vi "ReadCluster.vi"(1 "reference":refnum<vi>) -> (0 "Cluster":T6)   [LabVIEW 2013]
uses:
  <vilib>/Utility/miscctls.llb/LVBoundsTypeDef.ctl
  <vilib>/Utility/miscctls.llb/LVPositionTypeDef.ctl
  <vilib>/Utility/miscctls.llb/LVRectTypeDef.ctl
  <vilib>/Utility/miscctls.llb/LVDataSocketStatusTypeDef.ctl
  <vilib>/Utility/miscctls.llb/LVKeyNavTypeDef.ctl
panel:
  out "error out 72":errorcluster
  out "error out 71":errorcluster
  out "error out 70":errorcluster
  out "error out 69":errorcluster
  out "error out 68":errorcluster
  out "error out 67":errorcluster
  out "error out 66":errorcluster
  out "error out 65":errorcluster
  out "error out 64":errorcluster
  out "error out 63":errorcluster
  out "error out 62":errorcluster
  out "error out 61":errorcluster
  out "error out 60":errorcluster
  out "error out 59":errorcluster
  out "error out 58":errorcluster
  out "error out 57":errorcluster
  out "error out 56":errorcluster
  out "error out 55":errorcluster
  out "error out 54":errorcluster
  out "error out 53":errorcluster
  out "error out 52":errorcluster
  out "error out 51":errorcluster
  out "error out 50":errorcluster
  out "error out 49":errorcluster
  out "error out 48":errorcluster
  out "error out 47":errorcluster
  out "error out 46":errorcluster
  out "error out 45":errorcluster
  out "error out 44":errorcluster
  out "error out 43":errorcluster
  out "error out 42":errorcluster
  out "error out 41":errorcluster
  out "error out 40":errorcluster
  out "error out 39":errorcluster
  out "error out 38":errorcluster
  out "error out 37":errorcluster
  out "error out 36":errorcluster
  out "error out 35":errorcluster
  out "error out 34":errorcluster
  out "error out 33":errorcluster
  out "error out 32":errorcluster
  out "error out 31":errorcluster
  out "error out 30":errorcluster
  out "error out 29":errorcluster
  out "error out 28":errorcluster
  out "error out 27":errorcluster
  out "error out 26":errorcluster
  out "error out 25":errorcluster
  out "error out 24":errorcluster
  out "error out 23":errorcluster
  out "error out 22":errorcluster
  out "error out 21":errorcluster
  out "error out 20":errorcluster
  out "error out 19":errorcluster
  out "error out 18":errorcluster
  out "error out 17":errorcluster
  out "error out 16":errorcluster
  out "error out 15":errorcluster
  out "error out 14":errorcluster
  out "error out 13":errorcluster
  out "error out 12":errorcluster
  out "error out 11":errorcluster
  out "error out 10":errorcluster
  out "error out 9":errorcluster
  out "error out 8":errorcluster
  out "error out 7":errorcluster
  out "error out 6":errorcluster
  out "error out 5":errorcluster
  out "error out 4":errorcluster
  out "error out 3":errorcluster
  out "error out 2":errorcluster
  out "error out":errorcluster
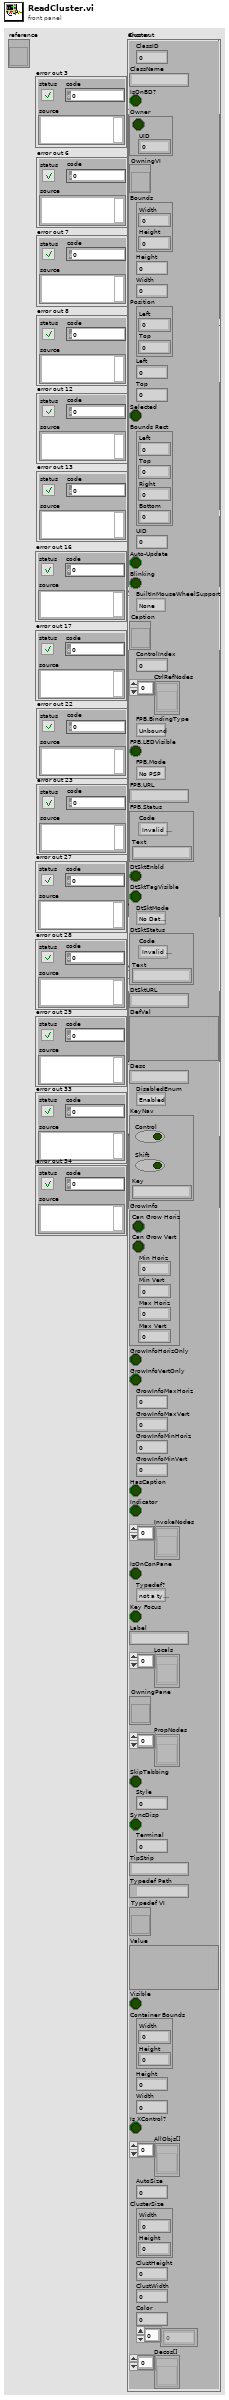
[diagram p1: front panel]
types:
  T1 = typedef "LVBoundsTypeDef.ctl" = cluster{"Width":u32, "Height":u32}
  T2 = typedef "LVPositionTypeDef.ctl" = cluster{"Left":i32, "Top":i32}
  T3 = typedef "LVRectTypeDef.ctl" = cluster{"Left":i16, "Top":i16, "Right":i16, "Bottom":i16}
  T4 = typedef "LVDataSocketStatusTypeDef.ctl" = cluster{"Code":enum32{"Invalid Status", "Unconnected", "Active", "Idle", "Error", "Connecting"}, "Text":string}
  T5 = typedef "LVKeyNavTypeDef.ctl" = cluster{"Control":bool, "Shift":bool, "Key":string}
  T6 = cluster{"ClassID":u32, "ClassName":string, "IsOnBD?":bool, "Owner":cluster{bool, "UID":i32}, "OwningVI":refnum<vi>, "Bounds":T1, "Height":u32, "Width":u32, "Position":T2, "Left":i32, "Top":i32, "Selected":bool, "Bounds Rect":T3, "UID":i32, "Auto-Update":bool, "Blinking":bool, "BuiltInMouseWheelSupport":enum16{"None", "On Hover", "On Key Focus", "On Hover or Key Focus"}, "Caption":refnum<vi>, "ControlIndex":i32, "CtrlRefNodes":refnum<vi>[], "FPB.BindingType":enum32{"Unbound", "Bound To PSP URL", "Bound To Variable Shortcut"}, "FPB.LEDVisible":bool, "FPB.Mode":enum32{"No PSP", "Read", "Write", "Write & Read"}, "FPB.URL":string, "FPB.Status":T4, "DtSktEnbld":bool, "DtSktTagVisible":bool, "DtSktMode":enum32{"No DataSocket", "Publish", "Subscribe", "Publish & Subscribe"}, "DtSktStatus":T4, "DtSktURL":string, "DefVal":variant, "Desc":string, "DisabledEnum":enum8{"Enabled", "Disabled", "Disabled and Grayed Out"}, "KeyNav":T5, "GrowInfo":cluster{"Can Grow Horiz":bool, "Can Grow Vert":bool, "Min Horiz":i16, "Min Vert":i16, "Max Horiz":i16, "Max Vert":i16}, "GrowInfoHorizOnly":bool, "GrowInfoVertOnly":bool, "GrowInfoMaxHoriz":i16, "GrowInfoMaxVert":i16, "GrowInfoMinHoriz":i16, "GrowInfoMinVert":i16, "HasCaption":bool, "Indicator":bool, "InvokeNodes":refnum<vi>[], "IsOnConPane":bool, "Typedef?":enum32{"not a typedef", "typedef", "strict typedef", "class private data"}, "Key Focus":bool, "Label":string, "Locals":refnum<vi>[], "OwningPane":refnum<vi>, "PropNodes":refnum<vi>[], "SkipTabbing":bool, "Style":u32, "SyncDisp":bool, "Terminal":i32, "TipStrip":string, "Typedef Path":path, "Typedef VI":refnum<vi>, "Value":variant, "Visible":bool, "Container Bounds":T1, "Height":u32, "Width":u32, "Is XControl?":bool, "AllObjs[]":refnum<vi>[], "AutoSize":u32, "ClusterSize":T1, "ClustHeight":u32, "ClustWidth":u32, "Color":u32, "Controls[]":i32[], "Decos[]":refnum<vi>[]}
  T7 = enum16{"None", "On Hover", "On Key Focus", "On Hover or Key Focus"}
  T8 = enum32{"No PSP", "Read", "Write", "Write & Read"}
  T9 = enum32{"Unbound", "Bound To PSP URL", "Bound To Variable Shortcut"}
  T10 = enum32{"No DataSocket", "Publish", "Subscribe", "Publish & Subscribe"}
  T11 = enum8{"Enabled", "Disabled", "Disabled and Grayed Out"}
  T12 = enum32{"not a typedef", "typedef", "strict typedef", "class private data"}
  T13 = cluster{"Can Grow Horiz":bool, "Can Grow Vert":bool, "Min Horiz":i16, "Min Vert":i16, "Max Horiz":i16, "Max Vert":i16}
  T14 = cluster{"ClassID":u32, "ClassName":string, "IsOnBD?":bool, "Cluster":cluster{bool, "UID":i32}, "OwningVI":refnum<vi>, "Bounds":T1, "Height":u32, "Width":u32, "Position":T2, "Left":i32, "Top":i32, "Selected":bool, "Bounds Rect":T3, "UID":i32, "Auto-Update":bool, "Blinking":bool, "BuiltInMouseWheelSupport":enum16{"None", "On Hover", "On Key Focus", "On Hover or Key Focus"}, "Caption":refnum<vi>, "ControlIndex":i32, "CtrlRefNodes":refnum<vi>[], "FPB.BindingType":enum32{"Unbound", "Bound To PSP URL", "Bound To Variable Shortcut"}, "FPB.LEDVisible":bool, "FPB.Mode":enum32{"No PSP", "Read", "Write", "Write & Read"}, "FPB.URL":string, "FPB.Status":T4, "DtSktEnbld":bool, "DtSktTagVisible":bool, "DtSktMode":enum32{"No DataSocket", "Publish", "Subscribe", "Publish & Subscribe"}, "DtSktStatus":T4, "DtSktURL":string, "DefVal":variant, "Desc":string, "DisabledEnum":enum8{"Enabled", "Disabled", "Disabled and Grayed Out"}, "KeyNav":T5, "GrowInfo":cluster{"Can Grow Horiz":bool, "Can Grow Vert":bool, "Min Horiz":i16, "Min Vert":i16, "Max Horiz":i16, "Max Vert":i16}, "GrowInfoHorizOnly":bool, "GrowInfoVertOnly":bool, "GrowInfoMaxHoriz":i16, "GrowInfoMaxVert":i16, "GrowInfoMinHoriz":i16, "GrowInfoMinVert":i16, "HasCaption":bool, "Indicator":bool, "InvokeNodes":refnum<vi>[], "IsOnConPane":bool, "Typedef?":enum32{"not a typedef", "typedef", "strict typedef", "class private data"}, "Key Focus":bool, "Text":string, "Locals":refnum<vi>[], "OwningPane":refnum<vi>, "PropNodes":refnum<vi>[], "SkipTabbing":bool, "Style":u32, "SyncDisp":bool, "UID":i32, "TipStrip":string, "Typedef Path":path, "Typedef VI":refnum<vi>, "Value":variant, "Visible":bool, "Container Bounds":T1, "Height":u32, "Width":u32, "Is XControl?":bool, "AllObjs[]":refnum<vi>[], "AutoSize":u32, "ClusterSize":T1, "ClustHeight":u32, "ClustWidth":u32, "Color":u32, i32[], "Decos[]":refnum<vi>[]}
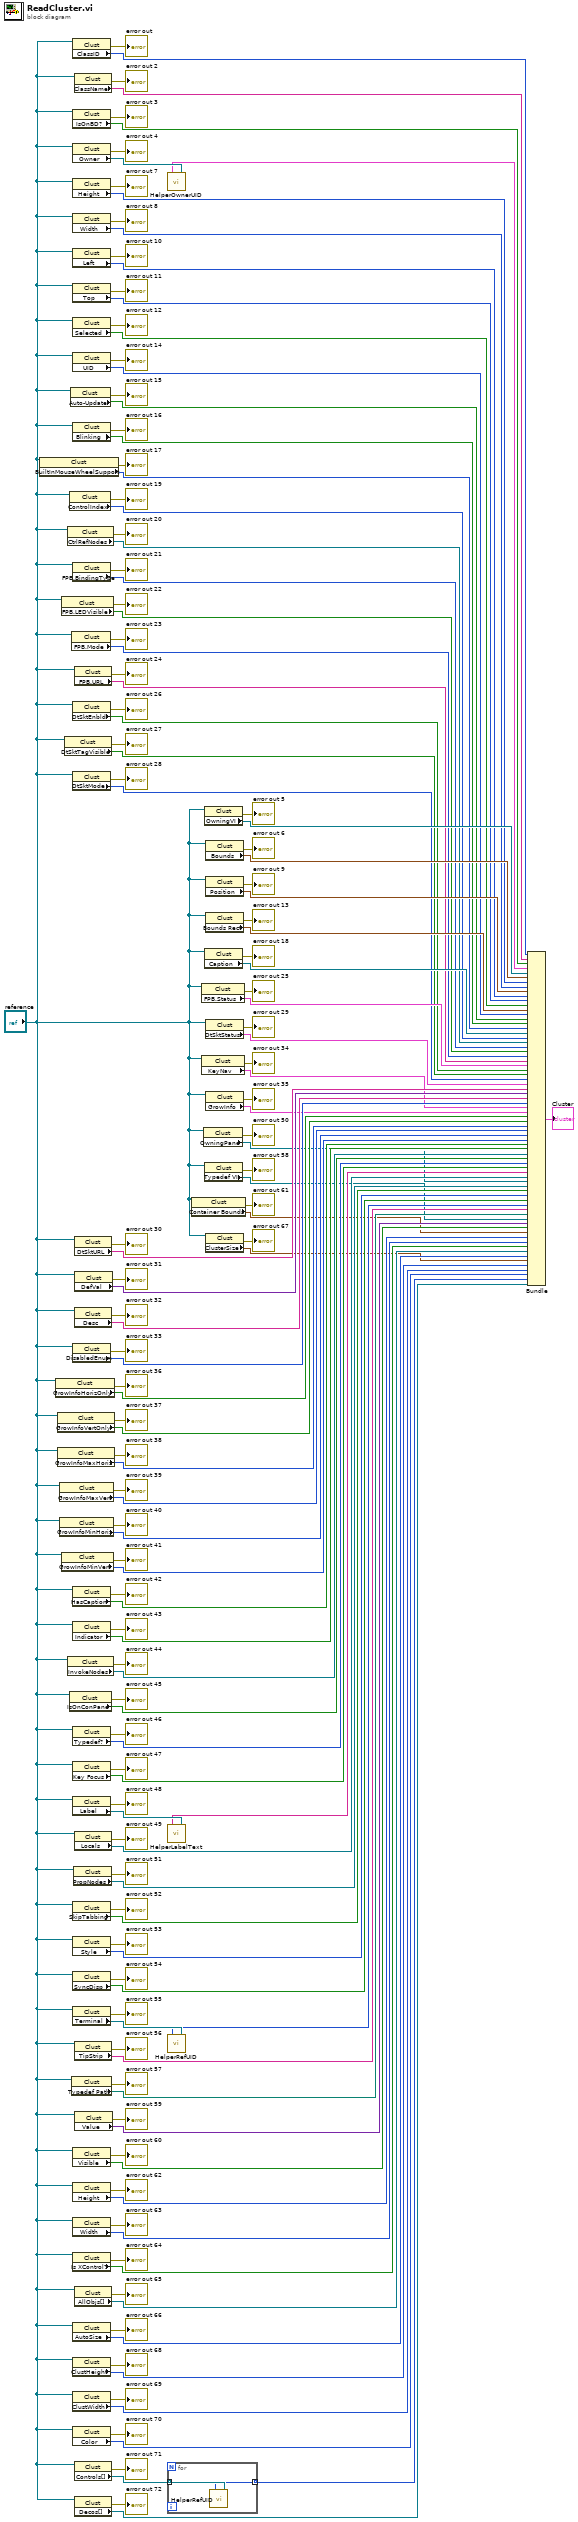
[diagram p0: block diagram]
diagram:
  n1 = property class="Clust"(reference="reference") -> (error out=→"error out 17":errorcluster, "BuiltInMouseWheelSupport"=w115:T7)  [unwired: 1 in, 1 out]
  n2 = property class="Clust"(reference="reference") -> (error out=→"error out 36":errorcluster, "GrowInfoHorizOnly"=w77:bool)  [unwired: 1 in, 1 out]
  n3 = property class="Clust"(reference="reference") -> (error out=→"error out 37":errorcluster, "GrowInfoVertOnly"=w75:bool)  [unwired: 1 in, 1 out]
  n4 = property class="Clust"(reference="reference") -> (error out=→"error out 38":errorcluster, "GrowInfoMaxHoriz"=w73:i16)  [unwired: 1 in, 1 out]
  n5 = property class="Clust"(reference="reference") -> (error out=→"error out 39":errorcluster, "GrowInfoMaxVert"=w71:i16)  [unwired: 1 in, 1 out]
  n6 = property class="Clust"(reference="reference") -> (error out=→"error out 40":errorcluster, "GrowInfoMinHoriz"=w69:i16)  [unwired: 1 in, 1 out]
  n7 = property class="Clust"(reference="reference") -> (error out=→"error out 22":errorcluster, "FPB.LEDVisible"=w105:bool)  [unwired: 1 in, 1 out]
  n8 = property class="Clust"(reference="reference") -> (error out=→"error out 41":errorcluster, "GrowInfoMinVert"=w67:i16)  [unwired: 1 in, 1 out]
  n9 = property class="Clust"(reference="reference") -> (error out=→"error out 27":errorcluster, "DtSktTagVisible"=w95:bool)  [unwired: 1 in, 1 out]
  n10 = property class="Clust"(reference="reference") -> (error out=→"error out 20":errorcluster, "CtrlRefNodes"=w109:refnum<vi>[])  [unwired: 1 in, 1 out]
  n11 = property class="Clust"(reference="reference") -> (error out=→"error out 44":errorcluster, "InvokeNodes"=w61:refnum<vi>[])  [unwired: 1 in, 1 out]
  n12 = property class="Clust"(reference="reference") -> (error out=→"error out 45":errorcluster, "IsOnConPane"=w59:bool)  [unwired: 1 in, 1 out]
  n13 = property class="Clust"(reference="reference") -> (error out=→"error out 19":errorcluster, "ControlIndex"=w111:i32)  [unwired: 1 in, 1 out]
  n14 = property class="Clust"(reference="reference") -> (error out=→"error out 15":errorcluster, "Auto-Update"=w119:bool)  [unwired: 1 in, 1 out]
  n15 = property class="Clust"(reference="reference") -> (error out=→"error out 23":errorcluster, "FPB.Mode"=w103:T8)  [unwired: 1 in, 1 out]
  n16 = property class="Clust"(reference="reference") -> (error out=→"error out 57":errorcluster, "Typedef Path"=w33:path)  [unwired: 1 in, 1 out]
  n17 = property class="Clust"(reference="reference") -> (error out=→"error out":errorcluster, "ClassID"=w148:u32)  [unwired: 1 in, 1 out]
  n18 = property class="Clust"(reference="reference") -> (error out=→"error out 3":errorcluster, "IsOnBD?"=w144:bool)  [unwired: 1 in, 1 out]
  n19 = property class="Clust"(reference="reference") -> (error out=→"error out 4":errorcluster, "Owner"=w142:refnum<vi>)  [unwired: 1 in, 1 out]
  n20 = property class="Clust"(reference="reference") -> (error out=→"error out 7":errorcluster, "Height"=w135:u32)  [unwired: 1 in, 1 out]
  n21 = property class="Clust"(reference="reference") -> (error out=→"error out 8":errorcluster, "Width"=w133:u32)  [unwired: 1 in, 1 out]
  n22 = property class="Clust"(reference="reference") -> (error out=→"error out 10":errorcluster, "Left"=w129:i32)  [unwired: 1 in, 1 out]
  n23 = property class="Clust"(reference="reference") -> (error out=→"error out 11":errorcluster, "Top"=w127:i32)  [unwired: 1 in, 1 out]
  n24 = property class="Clust"(reference="reference") -> (error out=→"error out 12":errorcluster, "Selected"=w125:bool)  [unwired: 1 in, 1 out]
  n25 = property class="Clust"(reference="reference") -> (error out=→"error out 14":errorcluster, "UID"=w121:i32)  [unwired: 1 in, 1 out]
  n26 = property class="Clust"(reference="reference") -> (error out=→"error out 16":errorcluster, "Blinking"=w117:bool)  [unwired: 1 in, 1 out]
  n27 = property class="Clust"(reference="reference") -> (error out=→"error out 21":errorcluster, "FPB.BindingType"=w107:T9)  [unwired: 1 in, 1 out]
  n28 = property class="Clust"(reference="reference") -> (error out=→"error out 26":errorcluster, "DtSktEnbld"=w97:bool)  [unwired: 1 in, 1 out]
  n29 = property class="Clust"(reference="reference") -> (error out=→"error out 28":errorcluster, "DtSktMode"=w93:T10)  [unwired: 1 in, 1 out]
  n30 = property class="Clust"(reference="reference") -> (error out=→"error out 33":errorcluster, "DisabledEnum"=w83:T11)  [unwired: 1 in, 1 out]
  n31 = property class="Clust"(reference="reference") -> (error out=→"error out 42":errorcluster, "HasCaption"=w65:bool)  [unwired: 1 in, 1 out]
  n32 = property class="Clust"(reference="reference") -> (error out=→"error out 43":errorcluster, "Indicator"=w63:bool)  [unwired: 1 in, 1 out]
  n33 = property class="Clust"(reference="reference") -> (error out=→"error out 46":errorcluster, "Typedef?"=w57:T12)  [unwired: 1 in, 1 out]
  n34 = property class="Clust"(reference="reference") -> (error out=→"error out 47":errorcluster, "Key Focus"=w55:bool)  [unwired: 1 in, 1 out]
  n35 = property class="Clust"(reference="reference") -> (error out=→"error out 48":errorcluster, "Label"=w53:refnum<vi>)  [unwired: 1 in, 1 out]
  n36 = property class="Clust"(reference="reference") -> (error out=→"error out 52":errorcluster, "SkipTabbing"=w44:bool)  [unwired: 1 in, 1 out]
  n37 = property class="Clust"(reference="reference") -> (error out=→"error out 53":errorcluster, "Style"=w42:u32)  [unwired: 1 in, 1 out]
  n38 = property class="Clust"(reference="reference") -> (error out=→"error out 54":errorcluster, "SyncDisp"=w40:bool)  [unwired: 1 in, 1 out]
  n39 = property class="Clust"(reference="reference") -> (error out=→"error out 55":errorcluster, "Terminal"=w38:refnum<vi>)  [unwired: 1 in, 1 out]
  n40 = property class="Clust"(reference="reference") -> (error out=→"error out 60":errorcluster, "Visible"=w27:bool)  [unwired: 1 in, 1 out]
  n41 = property class="Clust"(reference="reference") -> (error out=→"error out 62":errorcluster, "Height"=w23:u32)  [unwired: 1 in, 1 out]
  n42 = property class="Clust"(reference="reference") -> (error out=→"error out 63":errorcluster, "Width"=w21:u32)  [unwired: 1 in, 1 out]
  n43 = property class="Clust"(reference="reference") -> (error out=→"error out 64":errorcluster, "Is XControl?"=w19:bool)  [unwired: 1 in, 1 out]
  n44 = property class="Clust"(reference="reference") -> (error out=→"error out 66":errorcluster, "AutoSize"=w15:u32)  [unwired: 1 in, 1 out]
  n45 = property class="Clust"(reference="reference") -> (error out=→"error out 68":errorcluster, "ClustHeight"=w11:u32)  [unwired: 1 in, 1 out]
  n46 = property class="Clust"(reference="reference") -> (error out=→"error out 69":errorcluster, "ClustWidth"=w9:u32)  [unwired: 1 in, 1 out]
  n47 = property class="Clust"(reference="reference") -> (error out=→"error out 70":errorcluster, "Color"=w7:u32)  [unwired: 1 in, 1 out]
  n48 = property class="Clust"(reference="reference") -> (error out=→"error out 51":errorcluster, "PropNodes"=w46:refnum<vi>[])  [unwired: 1 in, 1 out]
  n49 = property class="Clust"(reference="reference") -> (error out=→"error out 2":errorcluster, "ClassName"=w146:string)  [unwired: 1 in, 1 out]
  n50 = property class="Clust"(reference="reference") -> (error out=→"error out 24":errorcluster, "FPB.URL"=w101:string)  [unwired: 1 in, 1 out]
  n51 = property class="Clust"(reference="reference") -> (error out=→"error out 30":errorcluster, "DtSktURL"=w89:string)  [unwired: 1 in, 1 out]
  n52 = property class="Clust"(reference="reference") -> (error out=→"error out 32":errorcluster, "Desc"=w85:string)  [unwired: 1 in, 1 out]
  n53 = property class="Clust"(reference="reference") -> (error out=→"error out 49":errorcluster, "Locals"=w50:refnum<vi>[])  [unwired: 1 in, 1 out]
  n54 = property class="Clust"(reference="reference") -> (error out=→"error out 56":errorcluster, "TipStrip"=w35:string)  [unwired: 1 in, 1 out]
  n55 = property class="Clust"(reference="reference") -> (error out=→"error out 65":errorcluster, "AllObjs[]"=w17:refnum<vi>[])  [unwired: 1 in, 1 out]
  n56 = property class="Clust"(reference="reference") -> (error out=→"error out 71":errorcluster, "Controls[]"=w5:refnum<vi>[])  [unwired: 1 in, 1 out]
  n57 = property class="Clust"(reference="reference") -> (error out=→"error out 72":errorcluster, "Decos[]"=w2:refnum<vi>[])  [unwired: 1 in, 1 out]
  n58 = property class="Clust"(reference="reference") -> (error out=→"error out 31":errorcluster, "DefVal"=w87:variant)  [unwired: 1 in, 1 out]
  n59 = property class="Clust"(reference="reference") -> (error out=→"error out 59":errorcluster, "Value"=w29:variant)  [unwired: 1 in, 1 out]
  n60 = call "HelperOwnerUID.vi"("Generic in"=w142) -> ("Cluster"=w141:cluster{bool, "UID":i32})
  n61 = call "HelperLabelText.vi"("Text in"=w53) -> ("Text"=w52:string)
  n62 = call "HelperRefUID.vi"("Text in"=w38) -> ("UID"=w37:i32)
  n63 = for {
    tunnel: w5 -> [w152] mode=indexing
    tunnel: [w151] -> w4 mode=indexing
    n64 = call "HelperRefUID.vi"("Text in"=w152) -> ("UID"=w151:i32)
  }
  n65 = property class="Clust"(reference="reference") -> (error out=→"error out 61":errorcluster, "Container Bounds"=w25:T1)  [unwired: 1 in, 1 out]
  n66 = property class="Clust"(reference="reference") -> (error out=→"error out 25":errorcluster, "FPB.Status"=w99:T4)  [unwired: 1 in, 1 out]
  n67 = property class="Clust"(reference="reference") -> (error out=→"error out 34":errorcluster, "KeyNav"=w81:T5)  [unwired: 1 in, 1 out]
  n68 = property class="Clust"(reference="reference") -> (error out=→"error out 50":errorcluster, "OwningPane"=w48:refnum<vi>)  [unwired: 1 in, 1 out]
  n69 = property class="Clust"(reference="reference") -> (error out=→"error out 5":errorcluster, "OwningVI"=w139:refnum<vi>)  [unwired: 1 in, 1 out]
  n70 = property class="Clust"(reference="reference") -> (error out=→"error out 18":errorcluster, "Caption"=w113:refnum<vi>)  [unwired: 1 in, 1 out]
  n71 = property class="Clust"(reference="reference") -> (error out=→"error out 58":errorcluster, "Typedef VI"=w31:refnum<vi>)  [unwired: 1 in, 1 out]
  n72 = property class="Clust"(reference="reference") -> (error out=→"error out 6":errorcluster, "Bounds"=w137:T1)  [unwired: 1 in, 1 out]
  n73 = property class="Clust"(reference="reference") -> (error out=→"error out 9":errorcluster, "Position"=w131:T2)  [unwired: 1 in, 1 out]
  n74 = property class="Clust"(reference="reference") -> (error out=→"error out 13":errorcluster, "Bounds Rect"=w123:T3)  [unwired: 1 in, 1 out]
  n75 = property class="Clust"(reference="reference") -> (error out=→"error out 29":errorcluster, "DtSktStatus"=w91:T4)  [unwired: 1 in, 1 out]
  n76 = property class="Clust"(reference="reference") -> (error out=→"error out 35":errorcluster, "GrowInfo"=w79:T13)  [unwired: 1 in, 1 out]
  n77 = property class="Clust"(reference="reference") -> (error out=→"error out 67":errorcluster, "ClusterSize"=w13:T1)  [unwired: 1 in, 1 out]
  n78 = Bundle("ClassID"=w148, "ClassName"=w146, "IsOnBD?"=w144, "Cluster"=w141, "OwningVI"=w139, "Bounds"=w137, "Height"=w135, "Width"=w133, "Position"=w131, "Left"=w129, "Top"=w127, "Selected"=w125, "Bounds Rect"=w123, "UID"=w121, "Auto-Update"=w119, "Blinking"=w117, "BuiltInMouseWheelSupport"=w115, "Caption"=w113, "ControlIndex"=w111, "CtrlRefNodes"=w109, "FPB.BindingType"=w107, "FPB.LEDVisible"=w105, "FPB.Mode"=w103, "FPB.URL"=w101, "FPB.Status"=w99, "DtSktEnbld"=w97, "DtSktTagVisible"=w95, "DtSktMode"=w93, "DtSktStatus"=w91, "DtSktURL"=w89, "DefVal"=w87, "Desc"=w85, "DisabledEnum"=w83, "KeyNav"=w81, "GrowInfo"=w79, "GrowInfoHorizOnly"=w77, "GrowInfoVertOnly"=w75, "GrowInfoMaxHoriz"=w73, "GrowInfoMaxVert"=w71, "GrowInfoMinHoriz"=w69, "GrowInfoMinVert"=w67, "HasCaption"=w65, "Indicator"=w63, "InvokeNodes"=w61, "IsOnConPane"=w59, "Typedef?"=w57, "Key Focus"=w55, "Text"=w52, "Locals"=w50, "OwningPane"=w48, "PropNodes"=w46, "SkipTabbing"=w44, "Style"=w42, "SyncDisp"=w40, "UID"=w37, "TipStrip"=w35, "Typedef Path"=w33, "Typedef VI"=w31, "Value"=w29, "Visible"=w27, "Container Bounds"=w25, "Height"=w23, "Width"=w21, "Is XControl?"=w19, "AllObjs[]"=w17, "AutoSize"=w15, "ClusterSize"=w13, "ClustHeight"=w11, "ClustWidth"=w9, "Color"=w7, w4, "Decos[]"=w2) -> (→"Cluster":T14)  [unwired: 1 in]
